vi "create_or_extend_task.vi"(8 "error in (no error)":errorcluster, 11 "DAQmxWriteSignals in":refnum<class "SignalWriterDL090202DAQmx.lvclass">) -> (0 "error out":errorcluster, 2 "output task":refnum<k21>, 3 "DAQmxWriteSignals out":refnum<class "SignalWriterDL090202DAQmx.lvclass">, 4 "newly created?":bool)   [LabVIEW 2010, in "SignalWriterDL090202DAQmx.lvclass"]
uses:
  SignalWriterDL090202DAQmx.lvclass
  common/clusters/counter_settings_cluster.ctl
  <vilib>/DAQmx/create/channels.llb/DAQmx Create Channel (AO-Voltage-Basic).vi
  <vilib>/DAQmx/create/channels.llb/DAQmx Create Channel (DO-Digital Output).vi
  <vilib>/DAQmx/create/channels.llb/DAQmx Create Channel (CO-Pulse Generation-Ticks).vi
  <vilib>/DAQmx/configure/timing.llb/DAQmx Timing (Implicit).vi
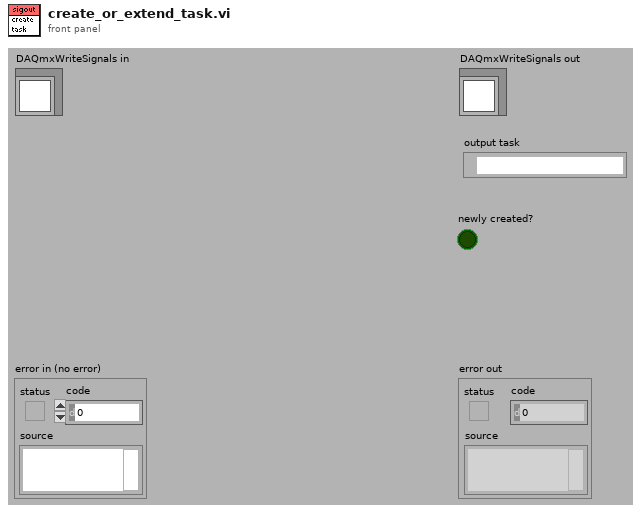
[diagram p1: front panel]
types:
  T1 = typedef "counter_settings_cluster.ctl" = cluster{"offset cycles":i32, "high cycles":i32, "low cycles":i32}
  T2 = typedef "SignalWriterDL090202DAQmx.lvclass/output_type_enum.ctl" = enum16{"analog", "digital (U8)", "digital (U16)", "digital (U32)"}
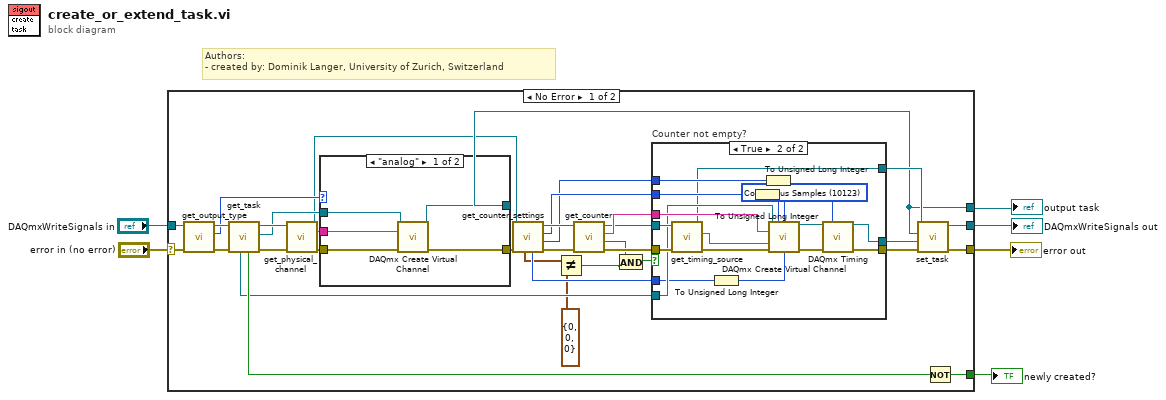
[diagram p0: block diagram]
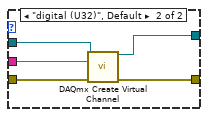
[diagram p3: hidden frame]
diagram:
  # "Authors: \n- created by: Dominik Langer, University of Zurich, Switzerland"
  n1 = case shown="No Error" "error in (no error)" {
    selector: "error in (no error)" -> [w31 w73]
    tunnel: [w38 w73] -> w4
    tunnel: [w37 w72] -> w3
    tunnel: "DAQmxWriteSignals in" -> [w28 w72]
    tunnel: [w20 _] -> w2
    tunnel: [w32 _] -> w1
    frame No Error {
      n2 = call-dynamic "get_output_type.vi"("error in (no error)"=w31, "DAQmxWriteSignals.lvclass in"=w28) -> ("error out"=w30:errorcluster, "output type"=w27:T2, "DAQmxWriteSignals.lvclass out"=w29:refnum<class "SignalWriterDL090202DAQmx.lvclass">)  [unwired: 7 out]
      n3 = call-dynamic "get_task.vi"("error in (no error)"=w30, "DAQmxWriteSignals in"=w29) -> ("error out"=w36:errorcluster, "writer task"=w34:refnum<k21>, "DAQmxWriteSignals out"=w35:refnum<class "SignalWriterDL090202DAQmx.lvclass">, "found?"=w33:bool, "counter task"=w21:refnum<k21>)  [unwired: 5 out]
      n4 = call-dynamic "get_physical_channel.vi"("error in (no error)"=w36, "DAQmxWriteSignals.lvclass in"=w35) -> ("error out"=w39:errorcluster, "physical channel"=w40:tag, "DAQmxWriteSignals.lvclass out"=w16:refnum<class "SignalWriterDL090202DAQmx.lvclass">)  [unwired: 7 out]
      n5 = case shown="\"analog\"" w27 {
        tunnel: w40 -> [w66 w69]
        tunnel: w39 -> [w65 w71]
        tunnel: [w64 w70] -> w17
        tunnel: [w63 w67] -> w20
        tunnel: w34 -> [w62 w68]
        frame "analog" {
          n6 = call-poly <vilib>:"DAQmx Create Virtual Channel.vi"("task in"=w62, "physical channels"=w66, "error in"=w65) -> ("task out"=w63:refnum<k21>, "error out"=w64:errorcluster)  [unwired: 6 in, 5 out]
        }
        frame "digital (U32)", Default {
          n7 = call-poly <vilib>:"DAQmx Create Virtual Channel.vi"("task in"=w68, "lines"=w69, "error in"=w71) -> ("task out"=w67:refnum<k21>, "error out"=w70:errorcluster)  [unwired: 2 in, 9 out]
        }
      }
      n8 = call-dynamic "get_counter_settings.vi"("error in (no error)"=w17, "GenericSignalWriter in"=w16) -> ("error out"=w18:errorcluster, "low ticks"=w13:i32, "high ticks"=w14:i32, "GenericSignalWriter out"=w15:refnum<class "SignalWriterDL090202DAQmx.lvclass">, "offset ticks"=w12:i32, "counter"=w11:T1)  [unwired: 4 in]
      n9 = Not Equal?(x=w11, y=T1 {"offset cycles"=0, "high cycles"=0, "low cycles"=0} ("counter")) -> (x != y?=w9:bool)
      n10 = call-dynamic "get_counter.vi"("error in (no error)"=w18, "SignalWriterDL090202DAQmx in"=w15) -> ("error out"=w25:errorcluster, "not empty?"=w8:bool, "counter"=w24:tag, "SignalWriterDL090202DAQmx out"=w23:refnum<class "SignalWriterDL090202DAQmx.lvclass">)  [unwired: 6 in]
      n11 = And(x=w8, y=w9) -> (x .and. y?=w7:bool)
      n12 = case "Counter not empty?" shown="True" w7 {
        tunnel: [w43 w46] -> w26
        tunnel: w25 -> [w43 w57]
        tunnel: w24 -> [_ w61]
        tunnel: w23 -> [w42 w56]
        tunnel: [w42 w51] -> w22
        tunnel: w21 -> [w41 w54]
        tunnel: [w41 w44] -> w19
        tunnel: w14 -> [_ w53]
        tunnel: w13 -> [_ w52]
        tunnel: w12 -> [_ w49]
        frame False {
        }
        frame True {
          w48 = 10123 items=["Finite Samples"=10178, "Continuous Samples"=10123, "Hardware Timed Single Point"=12522] ("sample mode")
          n13 = call-dynamic "get_timing_source.vi"("error in (no error)"=w57, "DAQmxWriteSignals.lvclass in"=w56) -> ("error out"=w50:errorcluster, "timing source"=w55:tag, "DAQmxWriteSignals.lvclass out"=w51:refnum<class "SignalWriterDL090202DAQmx.lvclass">)  [unwired: 7 in]
          n14 = To Unsigned Long Integer(number=w49) -> (unsigned 32bit integer=w60:u32)
          n15 = To Unsigned Long Integer(number=w53) -> (unsigned 32bit integer=w58:u32)
          n16 = To Unsigned Long Integer(number=w52) -> (unsigned 32bit integer=w59:u32)
          n17 = call-poly <vilib>:"DAQmx Create Virtual Channel.vi"("task in"=w54, "high ticks"=w58, "low ticks"=w59, "counter"=w61, "source of ticks"=w55, "error in"=w50, "initial delay"=w60) -> ("task out"=w45:refnum<k21>, "error out"=w47:errorcluster)  [unwired: 7 in]
          n18 = call-poly <vilib>:"DAQmx Timing.vi"("task/channels in"=w45, "sample mode"=w48, "error in"=w47) -> ("task out"=w44:refnum<k21>, "error out"=w46:errorcluster)  [unwired: 11 in]
        }
      }
      n19 = call-dynamic "set_task.vi"("error in (no error)"=w26, "counter task"=w19, "output task"=w20, "DAQmxWriteSignals in"=w22) -> ("error out"=w38:errorcluster, "DAQmxWriteSignals out"=w37:refnum<class "SignalWriterDL090202DAQmx.lvclass">)  [unwired: 6 out]
      n20 = Not(x=w33) -> (.not. x?=w32:bool)
    }
    frame Error {
    }
  }
  "error out" <- w4
  "DAQmxWriteSignals out" <- w3
  "output task" <- w2
  "newly created?" <- w1
